vi "Periodic Tasks.vi"(8 "error in":errorcluster) -> ()   [LabVIEW 2019]
doc: "This VI runs in parallel to other tasks. It can contain as many user-defined periodic loops as you need. These can carry out PID or other sorts of timed response."
uses:
  <vilib>/Rock Robotics/WPI/Solenoid/WPI_SolenoidValue.ctl
  <vilib>/Rock Robotics/WPI/ThirdParty/Phoenix-LabVIEW/Motor Controller/Controls/CTRE_Phoenix_MotorControl_ControlMode.ctl
  GlobalRefnum.vi
  Joystick_Buttons.vi
  <vilib>/Rock Robotics/WPI/Solenoid/WPI_SolenoidSetEnum.vi
  Global Vars.vi
  <vilib>/Rock Robotics/WPI/ThirdParty/Phoenix-LabVIEW/Motor Controller/Get/CTRE_Phoenix_MotorController_GetSelectedSensorData.vi
  <vilib>/Rock Robotics/Network Tables/NT Read Number.vi
  <vilib>/Rock Robotics/Network Tables/NT Write Boolean.vi
  <vilib>/Rock Robotics/Network Tables/NT Write Number.vi
  <vilib>/Rock Robotics/WPI/Utilities/WPI_GetSetVariantRefNum.vi
  <vilib>/Rock Robotics/Network Tables/NT Write String.vi
  <vilib>/Rock Robotics/Network Tables/NT Write Numeric Array.vi
panel:
  out "TargetValid":bool
  in  "DriveK":dbl(slide)=0.26277372262773724 min=0.0 max=1.0 step=0.05 scale=0.0..20.0
  in  "AimDeadband":dbl min=0.0 max=10.0 step=0.25
  in  "MinSteerCommand":dbl(slide)=0.2717391304347826 min=0.0 max=0.5 step=0.05 scale=0.0..0.5
  in  "SteeringK":dbl(slide)=0.025362318840579712 min=0.0 max=0.25 step=0.01 scale=0.0..0.25
  out "Target X":dbl
  out "Target Y":dbl
  out "Target Spotted":bool
  in  "DriveScale":dbl(slide)=0.7556179775280899 min=0.25 max=1.0 step=0.1 scale=0.25..1.0
  in  "Steering Scale":dbl(slide)=0.6418539325842696 min=0.25 max=1.0 step=0.1 scale=0.25..1.0
  in  "Tab Control":T1(tab)
  out "Drive Mode":string
  out "Drive Direction":string
  out "Waveform Chart Velovity LM":i32(graph)
  out "Waveform Velocity RM Chart":i32(graph)
  out "Waveform Chart Position RM":i32(graph)
  out "Waveform Chart Position LM":i32(graph)
  out "Velocity RM":i32
  out "Position RM":i32
  out "Velocity LM":i32
  out "Position LM":i32
  out "Waveform Chart":i32(graph)
  out "Set Shooter Speed":dbl=15000.0 format="%#_13g"
  out "Velocity (Raw Sensor Units per 100 ms)":i32
  out "fireStatus":bool
  out "Intake Reverse?":bool
  out "Exterior Intake":i32(graph)
  out "Velocity (Raw Sensor Units per 100 ms) 2":i32
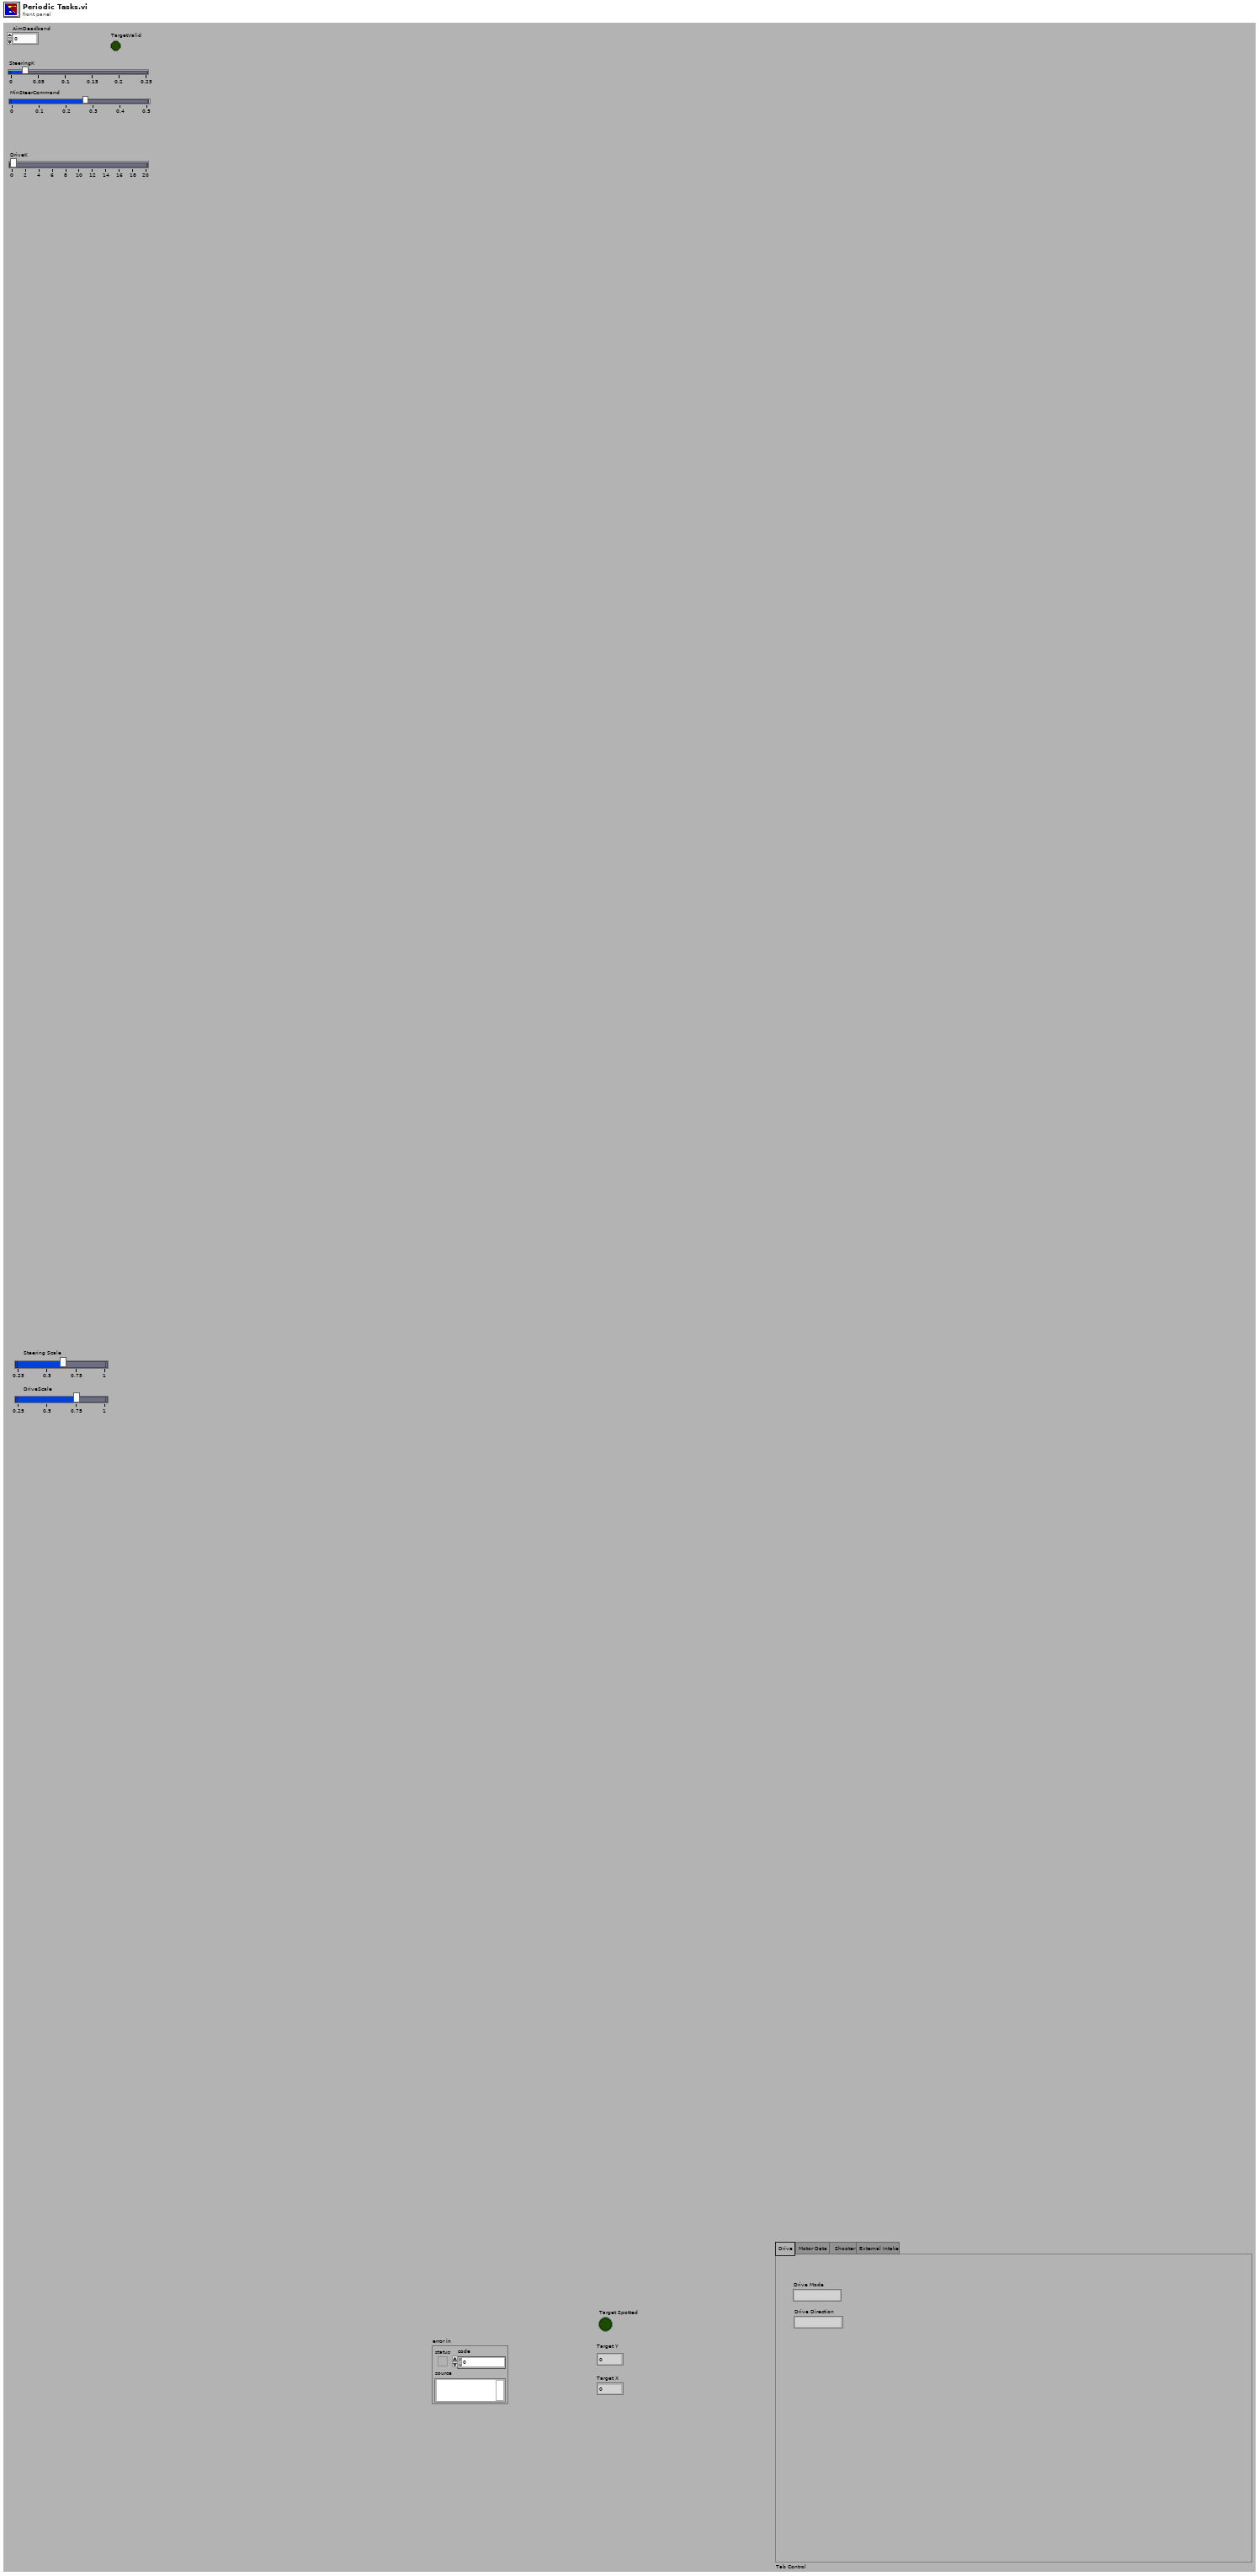
[diagram p1: front panel]
types:
  T1 = enum32{"Drive", "Motor Data", " Shooter", "External Intake"}
  T2 = typedef "WPI_RobotDriveDevRef.ctl" = cluster{"DevStatus":errorcluster, "Motors[]":T3[], "Square Inputs":bool, "Max Output":dbl}
  T3 = typedef "WPI_MotorControlDeviceRef.ctl" = cluster{"DeviceStatus":errorcluster, "Type":T4, "PWM":cluster{"PWM Channel":T5, "DeadBand":T6}, "CAN":cluster{"Device Number":u8, "SetOutput VI Ref":variant, "GetOutput VI Ref":variant, "Enable VI Ref":variant, "Disable VI Ref":variant, "Data":variant}, "Invert":bool, "DIO PWM":cluster{"PWM \"Enable\" Channel":T5, "DIOChannel":T7, "PWM Rate":dbl}}
  T4 = typedef "WPI_MotorControlType.ctl" = enum16{"PWM", "CAN", "DIO PWM"}
  T5 = typedef "FPGA_DIOPWMChannel.ctl" = enum8{"PWM 0", "PWM 1", "PWM 2", "PWM 3", "PWM 4", "PWM 5", "PWM 6", "PWM 7", "PWM 8", "PWM 9", "PWM MXP 0", "PWM MXP 1", "PWM MXP 2", "PWM MXP 3", "PWM MXP 4", "PWM MXP 5", "PWM MXP 6", "PWM MXP 7", "PWM MXP 8", "PWM MXP 9", "Invalid"}
  T6 = typedef "WPI_PWMDeadband.ctl" = cluster{"Name":string, "maxPositivePwm":i32, "minPositivePwm":i32, "centerPwm":i32, "maxNegativePwm":i32, "minNegativePwm":i32, "angularRange":u16}
  T7 = typedef "FPGA_DIOChannel.ctl" = enum8{"DIO 0", "DIO 1", "DIO 2", "DIO 3", "DIO 4", "DIO 5", "DIO 6", "DIO 7", "DIO 8", "DIO 9", "DIO MXP 0", "DIO MXP 1", "DIO MXP 2", "DIO MXP 3", "DIO MXP 4", "DIO MXP 5", "DIO MXP 6", "DIO MXP 7", "DIO MXP 8", "DIO MXP 9", "DIO MXP 10", "DIO MXP 11", "DIO MXP 12", "DIO MXP 13", "DIO MXP 14", "DIO MXP 15", "SPI Port CS1", "SPI Port CS2", "SPI Port CS3", "SPI Port MISO", "SPI Port MOSI", "Invalid"}
  T8 = typedef "CTRE_Phoenix_MotorControl_ControlMode.ctl" = u16
  T9 = typedef "WPI_SolenoidValue.ctl" = enum16{"Off", "On", "Forward", "Reverse"}
  T10 = typedef "WPI_SolenoidDevRef.ctl" = cluster{"DevStatus":errorcluster, "Pneumatics Control Module":u8, "Forward Solenoid Channel":T11, "Reverse Solenoid Channel":T11}
  T11 = typedef "WPI_SolenoidChannel.ctl" = enum8{"Solenoid 0", "Solenoid 1", "Solenoid 2", "Solenoid 3", "Solenoid 4", "Solenoid 5", "Solenoid 6", "Solenoid 7", "Invalid"}
  T12 = typedef "WPI_JoystickDevRef.ctl" = cluster{"Device":T13}
  T13 = typedef "WPI_JoystickDeviceEnum.ctl" = enum16{"USB 0", "USB 1", "USB 2", "USB 3", "USB 4", "USB 5"}
  T14 = cluster{"JoystickDevRef":T12, "RobotDriveDevRef":T2}
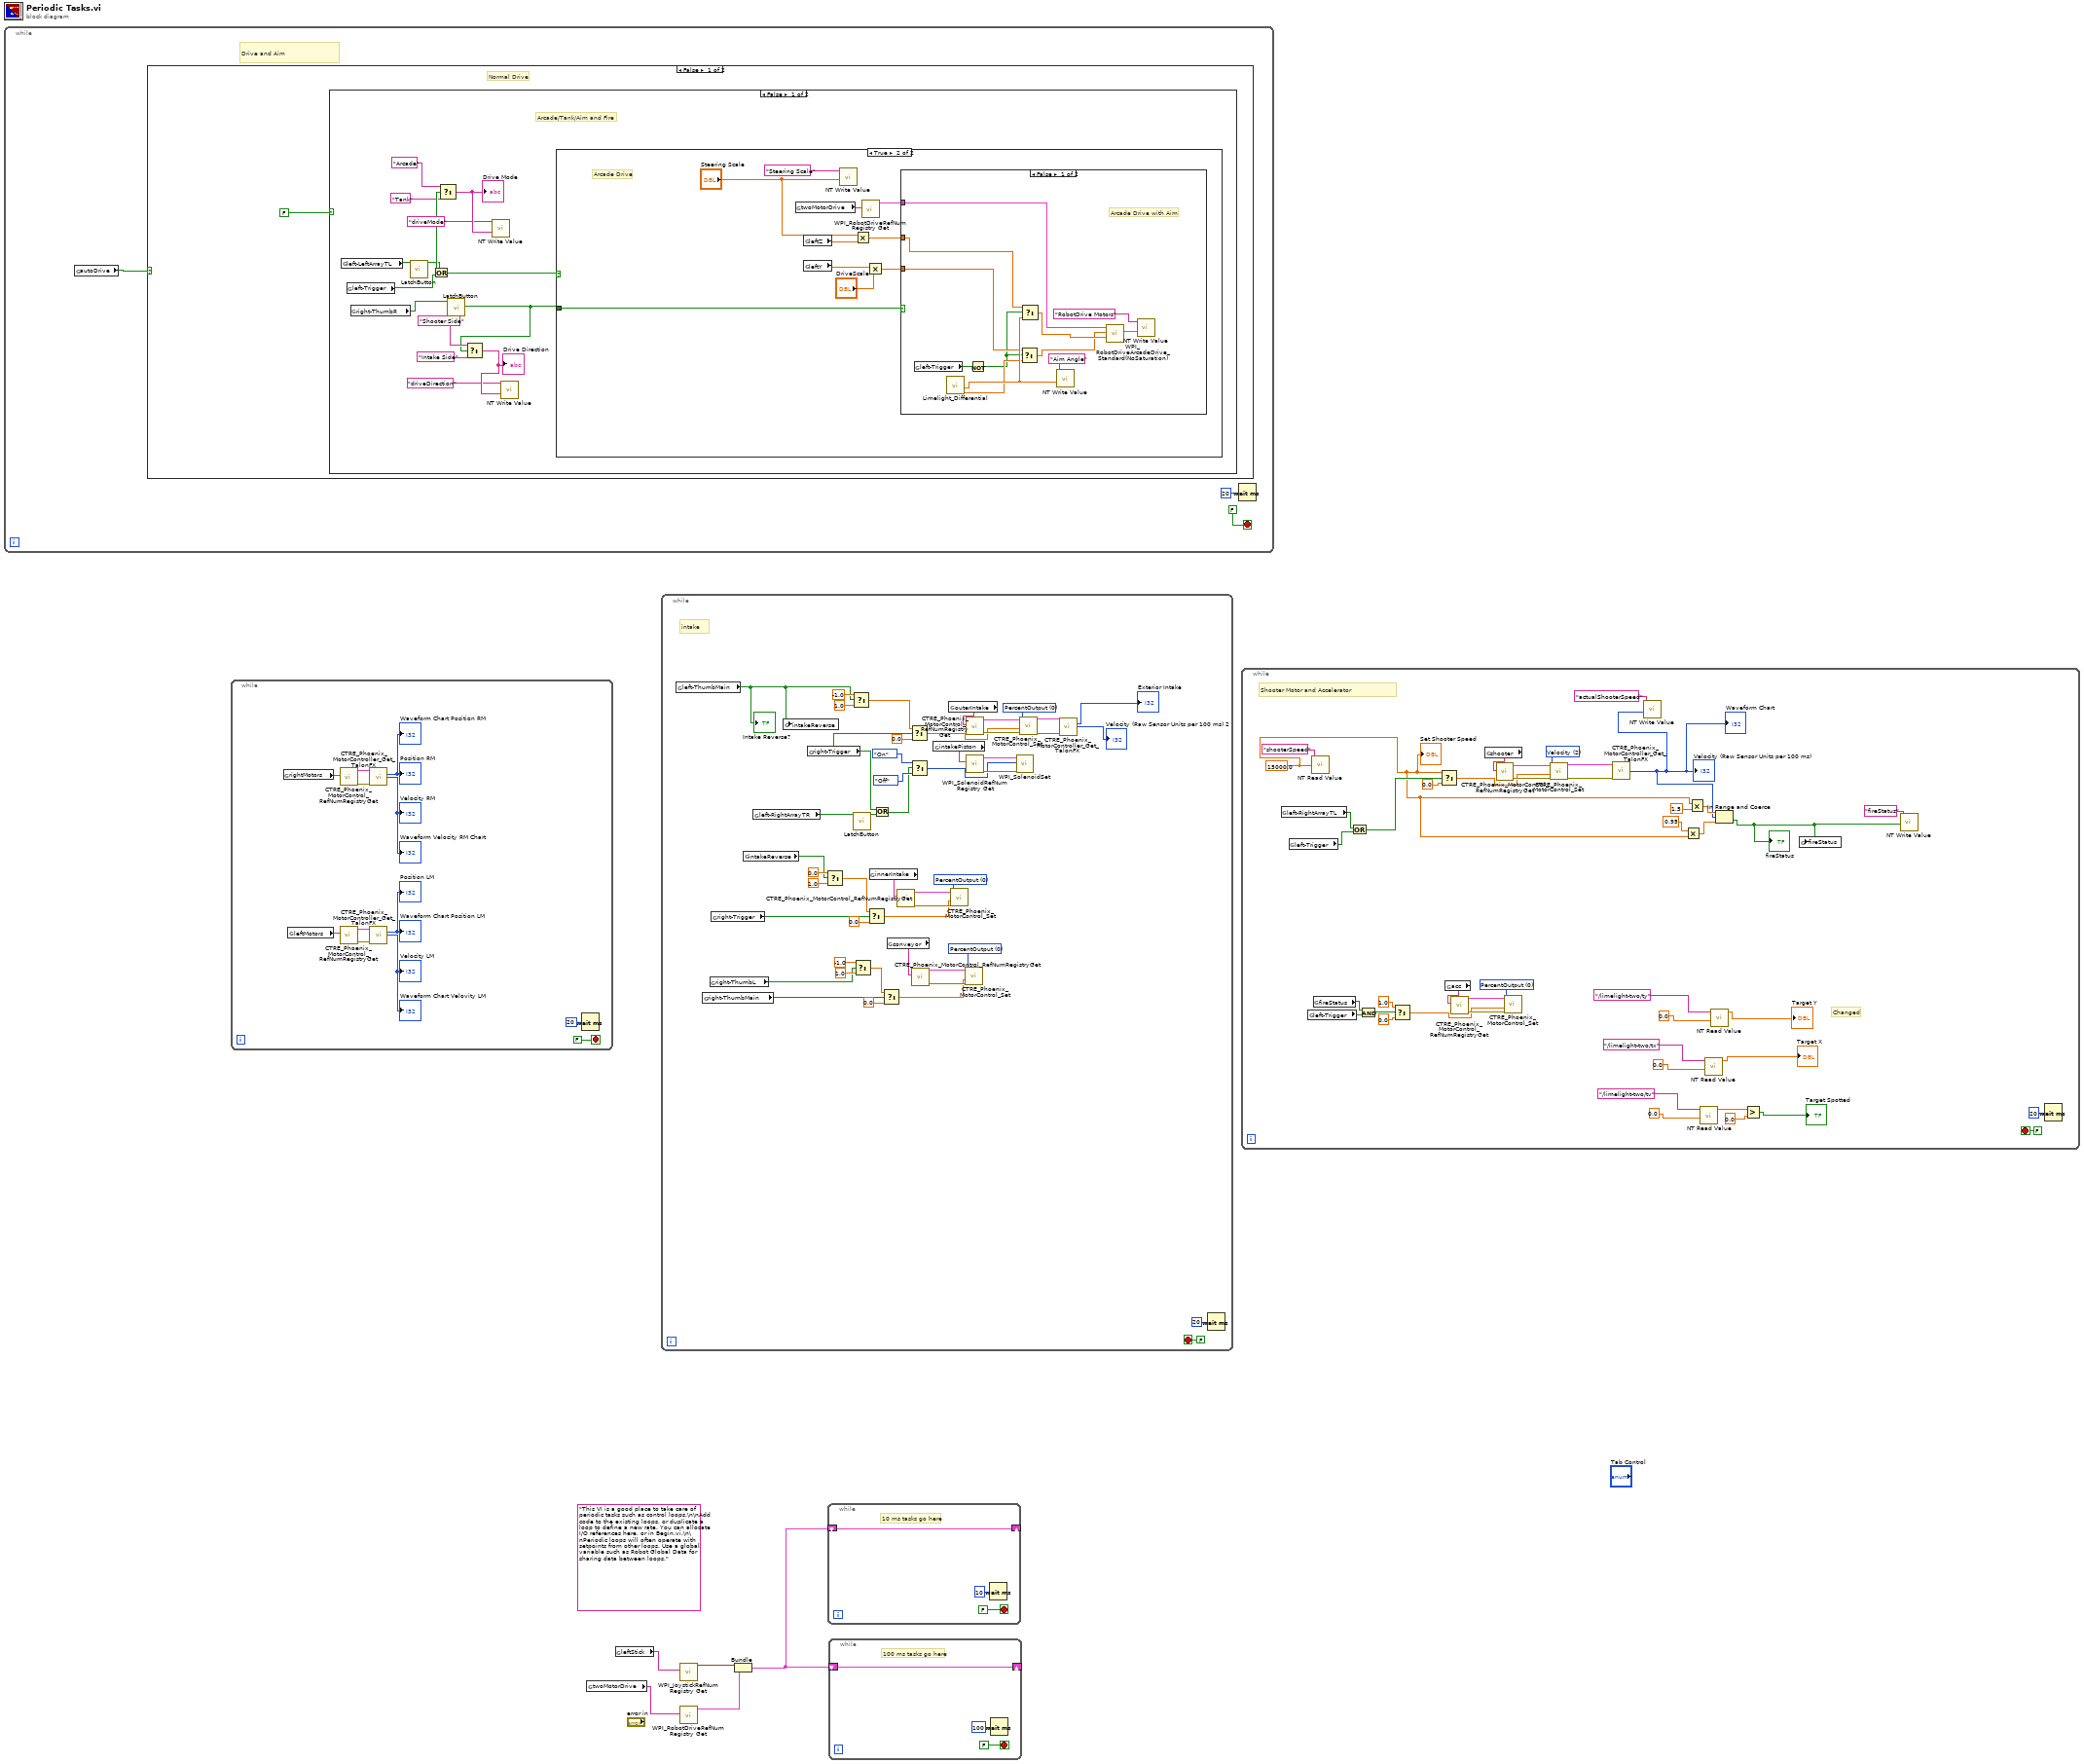
[diagram p0: block diagram]
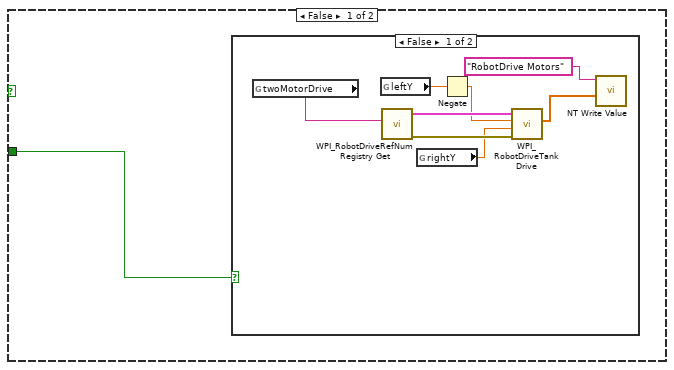
[diagram p2: hidden frame]
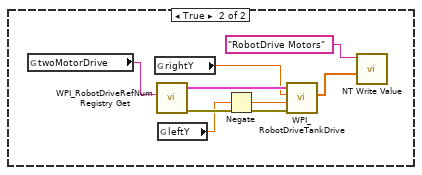
[diagram p3: hidden frame]
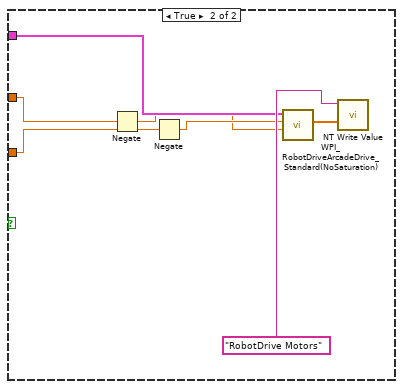
[diagram p4: hidden frame]
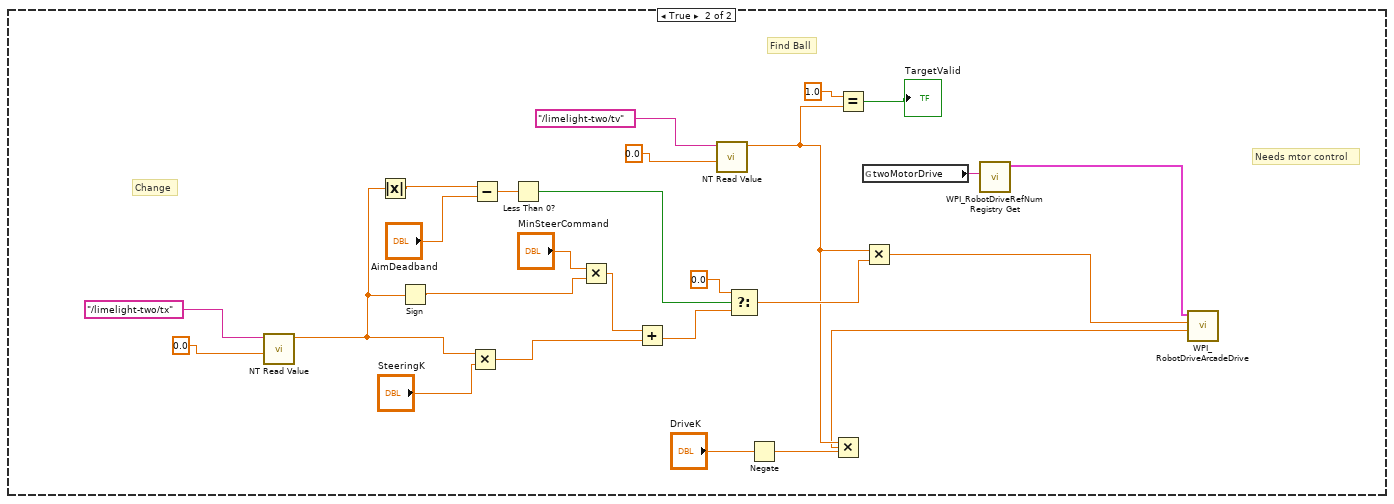
[diagram p5: hidden frame]
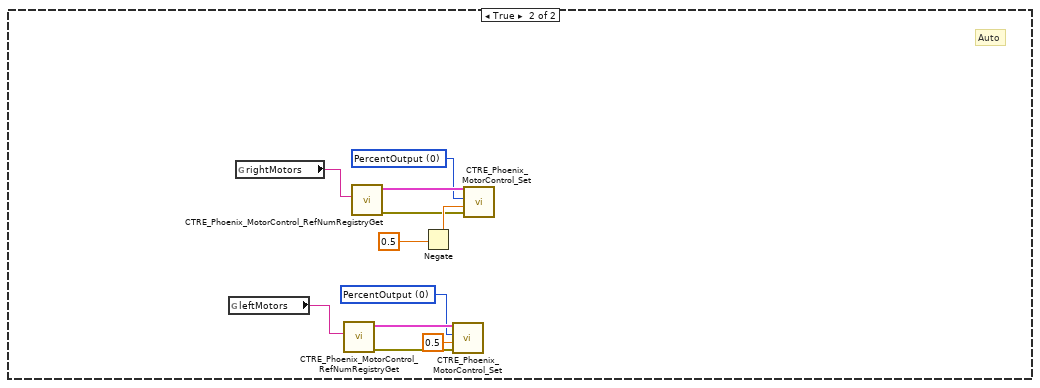
[diagram p6: hidden frame]
diagram:
  (unwired) "This VI is a good place to take care of periodic tasks such as control loops.\n\nAdd code to the existing loops, or duplicate a loop to define a new rate. You can allocate I/O references here, or in Begin.vi.\n\nPeriodic loops will often operate with setpoints from other loops. Use a global variable such as Robot Global Data for sharing data between loops."
  n1 = while {
    stop <- FALSE stop-if-true
    # "Drive and Aim"
    n2 = global read "Global Vars.vi" "autoDrive"() -> (w6:bool)
    n3 = case shown="False" w6 {
      frame False {
        # "Normal Drive"
        n4 = case shown="False" FALSE {
          frame False {
            # "Arcade/Tank/Aim and Fire"
            n5 = global read "Joystick_Buttons.vi" "left-LeftArrayTL"() -> (w17:bool)
            n6 = global read "Joystick_Buttons.vi" "left-Trigger"() -> (w23:bool)
            n7 = global read "Joystick_Buttons.vi" "right-ThumbR"() -> (w18:bool)
            n8 = call "LatchButton.vi"("Boolean In"=w17) -> ("Boolean Out"=w21:bool)  [unwired: 10 in]
            n9 = Or(x=w21, y=w23) -> (x .or. y?=w22:bool)
            n10 = Select(t="Arcade", s=w22, f="Tank") -> (s? t:f=w19:string)
            "Drive Mode" <- w19
            n11 = call "LatchButton.vi"("Boolean In"=w18) -> ("Boolean Out"=w10:bool)  [unwired: 10 in]
            n12 = Select(t="Shooter Side", s=w10, f="Intake Side") -> (s? t:f=w20:string)
            "Drive Direction" <- w20
            n13 = call-poly <vilib>:"NT Write Value.vi"("String"=w19, "Name"="driveMode") -> ()  [unwired: 9 in, 1 out]
            n14 = call-poly <vilib>:"NT Write Value.vi"("String"=w20, "Name"="driveDirection") -> ()  [unwired: 9 in, 1 out]
            n15 = case shown="True" w22 {
              tunnel: w10 -> [w24 w41]
              frame False {
                n16 = case shown="False" w24 {
                  frame False {
                    n17 = global read "GlobalRefnum.vi" "twoMotorDrive"() -> (w32:string)
                    n18 = global read "Joystick_Buttons.vi" "leftY"() -> (w29:dbl)
                    n19 = call <vilib>:"WPI_RobotDriveRefNum Registry Get.vi"("refnum name"=w32) -> ("error out"=w30:errorcluster, "RobotDriveDevRef"=w31:T2)  [unwired: 9 in]
                    n20 = global read "Joystick_Buttons.vi" "rightY"() -> (w28:dbl)
                    n21 = Negate(x=w29) -> (-x=w27:dbl)
                    n22 = call <vilib>:"WPI_RobotDriveTankDrive.vi"("error in (no error)"=w30, "Right axis value"=w28, "Left axis value"=w27, "RobotDriveDevRef"=w31) -> ("Motor Values"=w25:dbl[])  [unwired: 5 in, 2 out]
                    n23 = call-poly <vilib>:"NT Write Value.vi"("Numeric Array"=w25, "Name"="RobotDrive Motors") -> ()  [unwired: 9 in, 1 out]
                  }
                  frame True {
                    n24 = global read "GlobalRefnum.vi" "twoMotorDrive"() -> (w38:string)
                    n25 = global read "Joystick_Buttons.vi" "rightY"() -> (w35:dbl)
                    n26 = call <vilib>:"WPI_RobotDriveRefNum Registry Get.vi"("refnum name"=w38) -> ("error out"=w40:errorcluster, "RobotDriveDevRef"=w39:T2)  [unwired: 9 in]
                    n27 = global read "Joystick_Buttons.vi" "leftY"() -> (w37:dbl)
                    n28 = Negate(x=w37) -> (-x=w36:dbl)
                    n29 = call <vilib>:"WPI_RobotDriveTankDrive.vi"("error in (no error)"=w40, "Right axis value"=w36, "Left axis value"=w35, "RobotDriveDevRef"=w39) -> ("Motor Values"=w33:dbl[])  [unwired: 5 in, 2 out]
                    n30 = call-poly <vilib>:"NT Write Value.vi"("Numeric Array"=w33, "Name"="RobotDrive Motors") -> ()  [unwired: 9 in, 1 out]
                  }
                }
              }
              frame True {
                # "Arcade Drive"
                n31 = global read "GlobalRefnum.vi" "twoMotorDrive"() -> (w44:string)
                n32 = global read "Joystick_Buttons.vi" "leftZ"() -> (w43:dbl)
                n33 = global read "Joystick_Buttons.vi" "leftY"() -> (w42:dbl)
                n34 = call-poly <vilib>:"NT Write Value.vi"("Numeric"="Steering Scale", "Name"="Steering Scale") -> ()  [unwired: 9 in, 1 out]
                n35 = Multiply(x="Steering Scale", y=w43) -> (x*y=w47:dbl)
                n36 = call <vilib>:"WPI_RobotDriveRefNum Registry Get.vi"("refnum name"=w44) -> ("RobotDriveDevRef"=w46:T2)  [unwired: 1 in, 9 out]
                n37 = Multiply(x=w42, y="DriveScale") -> (x*y=w49:dbl)
                n38 = case shown="False" w41 {
                  tunnel: w49 -> [w60 w66]
                  tunnel: w47 -> [w59 w67]
                  tunnel: w46 -> [w56 w65]
                  frame False {
                    # "Arcade Drive with Aim"
                    n39 = global read "Joystick_Buttons.vi" "left-Trigger"() -> (w53:bool)
                    n40 = call "Limelight_Differential.vi"() -> ("DriveCommand"=w61:dbl, "SteerCommand"=w62:dbl)  [unwired: 8 in, 1 out]
                    n41 = Not(x=w53) -> (.not. x?=w58:bool)
                    n42 = Select(t=w60, s=w58, f=w61) -> (s? t:f=w51:dbl)
                    n43 = Select(t=w59, s=w58, f=w62) -> (s? t:f=w52:dbl)
                    n44 = call-poly <vilib>:"NT Write Value.vi"("Numeric"=w62, "Name"="Aim Angle") -> ()  [unwired: 9 in, 1 out]
                    n45 = call <vilib>:"WPI_RobotDriveArcadeDrive_Standard(NoSaturation).vi"("Y axis value"=w52, "X axis value"=w51, "RobotDriveDevRef"=w56) -> ("Motor Values"=w57:dbl[])  [unwired: 1 in, 7 out]
                    n46 = call-poly <vilib>:"NT Write Value.vi"("Numeric Array"=w57, "Name"="RobotDrive Motors") -> ()  [unwired: 9 in, 1 out]
                  }
                  frame True {
                    n47 = Negate(x=w67) -> (-x=w63:dbl)
                    n48 = Negate(x=w66) -> (-x=w64:dbl)
                    n49 = call <vilib>:"WPI_RobotDriveArcadeDrive_Standard(NoSaturation).vi"("Y axis value"=w63, "X axis value"=w64, "RobotDriveDevRef"=w65) -> ("Motor Values"=w69:dbl[])  [unwired: 1 in, 7 out]
                    n50 = call-poly <vilib>:"NT Write Value.vi"("Numeric Array"=w69, "Name"="RobotDrive Motors") -> ()  [unwired: 9 in, 1 out]
                  }
                }
              }
            }
          }
          frame True {
            # "Needs mtor control"
            # "Find Ball"
            # "Change"
            n51 = call-poly <vilib>:"NT Read Value.vi"("Default Value"=0.0, "Name"="/limelight-two/tx") -> ("Numeric"=w81:dbl)  [unwired: 8 in, 1 out]
            n52 = Absolute Value(x=w81) -> (abs(x)=w92:dbl)
            n53 = Sign(1:w81) -> (0:w82:dbl)
            n54 = Multiply(x=w81, y="SteeringK") -> (x*y=w89:dbl)
            n55 = Subtract(x=w92, y="AimDeadband") -> (x-y=w94:dbl)
            n56 = Less Than 0?(x=w94) -> (x < 0?=w74:bool)
            n57 = Multiply(x="MinSteerCommand", y=w82) -> (x*y=w91:dbl)
            n58 = Add(x=w91, y=w89) -> (x+y=w80:dbl)
            n59 = call-poly <vilib>:"NT Read Value.vi"("Default Value"=0.0, "Name"="/limelight-two/tv") -> ("Numeric"=w77:dbl)  [unwired: 8 in, 1 out]
            n60 = Select(t=0.0, s=w74, f=w80) -> (s? t:f=w84:dbl)
            n61 = Negate(x="DriveK") -> (-x=w75:dbl)
            n62 = Multiply(x=w77, y=w75) -> (x*y=w72:dbl)
            n63 = Equal?(x=1.0, y=w77) -> (x = y?=→"TargetValid":bool)
            n64 = global read "GlobalRefnum.vi" "twoMotorDrive"() -> (w71:string)
            n65 = Multiply(x=w77, y=w84) -> (x*y=w73:dbl)
            n66 = call <vilib>:"WPI_RobotDriveRefNum Registry Get.vi"("refnum name"=w71) -> ("RobotDriveDevRef"=w70:T2)  [unwired: 1 in, 9 out]
            n67 = call-poly <vilib>:"WPI_RobotDriveArcadeDrive.vi"("Y axis value"=w72, "X axis value"=w73, "RobotDriveDevRef"=w70) -> ()  [unwired: 6 in, 3 out]
          }
        }
      }
      frame True {
        w97 = T8 0 items=["PercentOutput"=0, "Position"=1, "Velocity"=2, "Current"=3, "Follower"=5, "MotionProfile"=6, "MotionMagic"=7, "MotionProfileArc"=10, "Disabled"=15] ("Control Mode")
        w99 = T8 0 items=["PercentOutput"=0, "Position"=1, "Velocity"=2, "Current"=3, "Follower"=5, "MotionProfile"=6, "MotionMagic"=7, "MotionProfileArc"=10, "Disabled"=15] ("Control Mode")
        # "Auto"
        n68 = global read "GlobalRefnum.vi" "leftMotors"() -> (w100:string)
        n69 = global read "GlobalRefnum.vi" "rightMotors"() -> (w105:string)
        n70 = call <vilib>:"CTRE_Phoenix_MotorControl_RefNumRegistryGet.vi"("refnum name"=w100) -> ("error out"=w102:errorcluster, "PhoenixMotorControlDevRef"=w101:T3)  [unwired: 9 in]
        n71 = call <vilib>:"CTRE_Phoenix_MotorControl_RefNumRegistryGet.vi"("refnum name"=w105) -> ("error out"=w104:errorcluster, "PhoenixMotorControlDevRef"=w103:T3)  [unwired: 9 in]
        n72 = Negate(x=0.5 ("Output")) -> (-x=w106:dbl)
        n73 = call <vilib>:"CTRE_Phoenix_MotorControl_Set.vi"("error in (no error)"=w102, "Output"=0.5, "Control Mode"=w97, "PhoenixMotorControlDevRef"=w101) -> ()  [unwired: 6 in, 2 out]
        n74 = call <vilib>:"CTRE_Phoenix_MotorControl_Set.vi"("error in (no error)"=w104, "Output"=w106, "Control Mode"=w99, "PhoenixMotorControlDevRef"=w103) -> ()  [unwired: 6 in, 2 out]
      }
    }
    n75 = Wait (ms)(milliseconds to wait=u32 20) -> ()  [unwired: 1 out]
  }
  n76 = while {
    stop <- FALSE stop-if-true
    n77 = global read "GlobalRefnum.vi" "rightMotors"() -> (w115:string)
    n78 = global read "GlobalRefnum.vi" "leftMotors"() -> (w116:string)
    n79 = call <vilib>:"CTRE_Phoenix_MotorControl_RefNumRegistryGet.vi"("refnum name"=w115) -> ("error out"=w111:errorcluster, "PhoenixMotorControlDevRef"=w112:T3)  [unwired: 9 in]
    n80 = call <vilib>:"CTRE_Phoenix_MotorControl_RefNumRegistryGet.vi"("refnum name"=w116) -> ("error out"=w113:errorcluster, "PhoenixMotorControlDevRef"=w114:T3)  [unwired: 9 in]
    n81 = call-poly <vilib>:"CTRE_Phoenix_MotorController_Get_TalonFX.vi"("PhoenixMotorControlDevRef"=w112, "error in"=w111) -> ("Position (Raw Sensor Units)"=→"Position RM" →"Waveform Chart Position RM":i32, "Velocity (Raw Sensor Units per 100 ms)"=→"Velocity RM" →"Waveform Velocity RM Chart":i32)  [unwired: 10 in, 2 out]
    n82 = call-poly <vilib>:"CTRE_Phoenix_MotorController_Get_TalonFX.vi"("PhoenixMotorControlDevRef"=w114, "error in"=w113) -> ("Position (Raw Sensor Units)"=→"Position LM" →"Waveform Chart Position LM":i32, "Velocity (Raw Sensor Units per 100 ms)"=→"Velocity LM" →"Waveform Chart Velovity LM":i32)  [unwired: 10 in, 2 out]
    n83 = Wait (ms)(milliseconds to wait=u32 20) -> ()  [unwired: 1 out]
  }
  n84 = global read "GlobalRefnum.vi" "twoMotorDrive"() -> (w1:string)
  n85 = global read "GlobalRefnum.vi" "leftStick"() -> (w2:string)
  n86 = while {
    stop <- FALSE stop-if-true
    w140 = T8 0 items=["PercentOutput"=0, "Position"=1, "Velocity"=2, "Current"=3, "Follower"=5, "MotionProfile"=6, "MotionMagic"=7, "MotionProfileArc"=10, "Disabled"=15] ("Control Mode")
    w146 = T8 0 items=["PercentOutput"=0, "Position"=1, "Velocity"=2, "Current"=3, "Follower"=5, "MotionProfile"=6, "MotionMagic"=7, "MotionProfileArc"=10, "Disabled"=15] ("Control Mode")
    w161 = T8 0 items=["PercentOutput"=0, "Position"=1, "Velocity"=2, "Current"=3, "Follower"=5, "MotionProfile"=6, "MotionMagic"=7, "MotionProfileArc"=10, "Disabled"=15] ("Control Mode")
    # "intake"
    n87 = global read "Joystick_Buttons.vi" "left-ThumbMain"() -> (w129:bool)
    "Intake Reverse?" <- w129
    n88 = global read "Joystick_Buttons.vi" "right-ThumbMain"() -> (w124:bool)
    n89 = global read "Joystick_Buttons.vi" "right-ThumbL"() -> (w133:bool)
    n90 = global read "Joystick_Buttons.vi" "right-Trigger"() -> (w123:bool)
    n91 = global read "Global Vars.vi" "intakeReverse"() -> (w126:bool)
    n92 = global read "Joystick_Buttons.vi" "left-RightArrayTR"() -> (w152:bool)
    n93 = global write "Global Vars.vi" "intakeReverse"(w129) -> ()
    n94 = global read "Joystick_Buttons.vi" "right-Trigger"() -> (w151:bool)
    n95 = Select(t=0.0, s=w126, f=1.0) -> (s? t:f=w125:dbl)
    n96 = Select(t=-1.0, s=w129, f=1.0) -> (s? t:f=w130:dbl)
    n97 = call "LatchButton.vi"("Boolean In"=w152) -> ("Boolean Out"=w150:bool)  [unwired: 10 in]
    n98 = Select(t=-1.0, s=w133, f=1.0) -> (s? t:f=w136:dbl)
    n99 = Select(t=w125, s=w123, f=0.0) -> (s? t:f=w143:dbl)
    n100 = global read "GlobalRefnum.vi" "innerIntake"() -> (w147:string)
    n101 = Or(x=w151, y=w150) -> (x .or. y?=w149:bool)
    n102 = Select(t=w136, s=w124, f=0.0) -> (s? t:f=w137:dbl)
    n103 = global read "GlobalRefnum.vi" "conveyor"() -> (w141:string)
    n104 = call <vilib>:"CTRE_Phoenix_MotorControl_RefNumRegistryGet.vi"("refnum name"=w147) -> ("error out"=w145:errorcluster, "PhoenixMotorControlDevRef"=w148:T3)  [unwired: 9 in]
    n105 = Select(t=w130, s=w151, f=0.0) -> (s? t:f=w159:dbl)
    n106 = Select(t=WPI_SolenoidValue."On" ("Value"), s=w149, f=WPI_SolenoidValue."Off" ("Value")) -> (s? t:f=w153:T9)
    n107 = call <vilib>:"CTRE_Phoenix_MotorControl_RefNumRegistryGet.vi"("refnum name"=w141) -> ("error out"=w139:errorcluster, "PhoenixMotorControlDevRef"=w142:T3)  [unwired: 9 in]
    n108 = global read "GlobalRefnum.vi" "intakePiston"() -> (w158:string)
    n109 = global read "GlobalRefnum.vi" "outerIntake"() -> (w162:string)
    n110 = call <vilib>:"CTRE_Phoenix_MotorControl_Set.vi"("error in (no error)"=w145, "Output"=w143, "Control Mode"=w146, "PhoenixMotorControlDevRef"=w148) -> ()  [unwired: 6 in, 2 out]
    n111 = call <vilib>:"CTRE_Phoenix_MotorControl_Set.vi"("error in (no error)"=w139, "Output"=w137, "Control Mode"=w140, "PhoenixMotorControlDevRef"=w142) -> ()  [unwired: 6 in, 2 out]
    n112 = call <vilib>:"CTRE_Phoenix_MotorControl_RefNumRegistryGet.vi"("refnum name"=w162) -> ("error out"=w163:errorcluster, "PhoenixMotorControlDevRef"=w164:T3)  [unwired: 9 in]
    n113 = call <vilib>:"WPI_SolenoidRefNum Registry Get.vi"("refnum name"=w158) -> ("error out"=w157:errorcluster, "SolenoidDevRef"=w156:T10)  [unwired: 9 in]
    n114 = call-poly <vilib>:"WPI_SolenoidSet.vi"("error in (no error)"=w157, "Value"=w153, "SolenoidDevRef"=w156) -> ()  [unwired: 7 in, 2 out]
    n115 = call <vilib>:"CTRE_Phoenix_MotorControl_Set.vi"("error in (no error)"=w163, "Output"=w159, "Control Mode"=w161, "PhoenixMotorControlDevRef"=w164) -> ("error out"=w121:errorcluster, "PhoenixMotorControlDevRef"=w122:T3)  [unwired: 6 in]
    n116 = call-poly <vilib>:"CTRE_Phoenix_MotorController_Get_TalonFX.vi"("PhoenixMotorControlDevRef"=w122, "error in"=w121) -> ("Position (Raw Sensor Units)"=→"Exterior Intake":i32, "Velocity (Raw Sensor Units per 100 ms)"=→"Velocity (Raw Sensor Units per 100 ms) 2":i32)  [unwired: 10 in, 2 out]
    n117 = Wait (ms)(milliseconds to wait=u32 20) -> ()  [unwired: 1 out]
  }
  n118 = call <vilib>:"WPI_JoystickRefNum Registry Get.vi"("refnum name"=w2) -> ("JoystickDevRef"=w5:T12)  [unwired: 1 in, 9 out]
  n119 = call <vilib>:"WPI_RobotDriveRefNum Registry Get.vi"("refnum name"=w1) -> ("RobotDriveDevRef"=w4:T2)  [unwired: 1 in, 9 out]
  n120 = Bundle("JoystickDevRef"=w5, "RobotDriveDevRef"=w4) -> (w3:T14)  [unwired: 1 out]
  n121 = while {
    shift-right: [w167] -> _
    shift-left: w3 -> [w167]
    stop <- FALSE stop-if-true
    # "10 ms tasks go here"
    n122 = Wait (ms)(milliseconds to wait=u32 10) -> ()  [unwired: 1 out]
  }
  n123 = while {
    shift-right: [w170] -> _
    shift-left: w3 -> [w170]
    stop <- FALSE stop-if-true
    # "100 ms tasks go here"
    n124 = Wait (ms)(milliseconds to wait=u32 100) -> ()  [unwired: 1 out]
  }
  n125 = while {
    stop <- FALSE stop-if-true
    w177 = 15000.0 ("Default Value")
    w206 = T8 0 items=["PercentOutput"=0, "Position"=1, "Velocity"=2, "Current"=3, "Follower"=5, "MotionProfile"=6, "MotionMagic"=7, "MotionProfileArc"=10, "Disabled"=15] ("Control Mode")
    w211 = T8 2 items=["PercentOutput"=0, "Position"=1, "Velocity"=2, "Current"=3, "Follower"=5, "MotionProfile"=6, "MotionMagic"=7, "MotionProfileArc"=10, "Disabled"=15] ("Control Mode")
    # "Changed"
    # "Shooter Motor and Accelerator"
    n126 = global read "Joystick_Buttons.vi" "left-RightArrayTL"() -> (w191:bool)
    n127 = global read "Joystick_Buttons.vi" "left-Trigger"() -> (w192:bool)
    n128 = global read "Joystick_Buttons.vi" "left-Trigger"() -> (w174:bool)
    n129 = call-poly <vilib>:"NT Read Value.vi"("Default Value"=w177, "Name"="shooterSpeed") -> ()  [unwired: 8 in, 2 out]
    n130 = global read "Global Vars.vi" "fireStatus"() -> (w176:bool)
    n131 = Or(x=w191, y=w192) -> (x .or. y?=w190:bool)
    n132 = And(x=w176, y=w174) -> (x .and. y?=w175:bool)
    n133 = Select(t=1.0, s=w175, f=0.0) -> (s? t:f=w204:dbl)
    n134 = Select(t=w177, s=w190, f=0.0) -> (s? t:f=w209:dbl)
    n135 = global read "GlobalRefnum.vi" "acc"() -> (w207:string)
    n136 = call <vilib>:"CTRE_Phoenix_MotorControl_RefNumRegistryGet.vi"("refnum name"=w207) -> ("error out"=w205:errorcluster, "PhoenixMotorControlDevRef"=w208:T3)  [unwired: 9 in]
    n137 = global read "GlobalRefnum.vi" "shooter"() -> (w212:string)
    n138 = call <vilib>:"CTRE_Phoenix_MotorControl_RefNumRegistryGet.vi"("refnum name"=w212) -> ("error out"=w213:errorcluster, "PhoenixMotorControlDevRef"=w214:T3)  [unwired: 9 in]
    n139 = call <vilib>:"CTRE_Phoenix_MotorControl_Set.vi"("error in (no error)"=w205, "Output"=w204, "Control Mode"=w206, "PhoenixMotorControlDevRef"=w208) -> ()  [unwired: 6 in, 2 out]
    n140 = call <vilib>:"CTRE_Phoenix_MotorControl_Set.vi"("error in (no error)"=w213, "Output"=w209, "Control Mode"=w211, "PhoenixMotorControlDevRef"=w214) -> ("error out"=w199:errorcluster, "PhoenixMotorControlDevRef"=w200:T3)  [unwired: 6 in]
    n141 = call-poly <vilib>:"CTRE_Phoenix_MotorController_Get_TalonFX.vi"("PhoenixMotorControlDevRef"=w200, "error in"=w199) -> ("Velocity (Raw Sensor Units per 100 ms)"=w173:i32)  [unwired: 10 in, 3 out]
    "Velocity (Raw Sensor Units per 100 ms)" <- w173
    "Waveform Chart" <- w173
    n142 = call-poly <vilib>:"NT Write Value.vi"("Numeric"=w173, "Name"="actualShooterSpeed") -> ()  [unwired: 9 in, 1 out]
    n143 = Multiply(x=0.95, y=w177) -> (x*y=w196:dbl)
    n144 = Multiply(x=w177, y=1.5) -> (x*y=w195:dbl)
    n145 = call-poly <vilib>:"NT Read Value.vi"("Default Value"=0.0, "Name"="/limelight-two/tv") -> ("Numeric"=w186:dbl)  [unwired: 8 in, 1 out]
    n146 = call-poly <vilib>:"NT Read Value.vi"("Default Value"=0.0, "Name"="/limelight-two/tx") -> ("Numeric"=→"Target X":dbl)  [unwired: 8 in, 1 out]
    n147 = call-poly <vilib>:"NT Read Value.vi"("Default Value"=0.0, "Name"="/limelight-two/ty") -> ("Numeric"=→"Target Y":dbl)  [unwired: 8 in, 1 out]
    n148 = In Range and Coerce(upper limit=w195, x=w173, lower limit=w196) -> (In Range?=w189:bool)  [unwired: 1 out]
    "fireStatus" <- w189
    n149 = Greater?(x=w186, y=0.0 ("Default Value")) -> (0:→"Target Spotted":bool)
    n150 = global write "Global Vars.vi" "fireStatus"(w189) -> ()
    n151 = call-poly <vilib>:"NT Write Value.vi"("Boolean"=w189, "Name"="fireStatus") -> ()  [unwired: 9 in, 1 out]
    n152 = Wait (ms)(milliseconds to wait=u32 20) -> ()  [unwired: 1 out]
    "Set Shooter Speed" <- w177
  }
